vi "Process.vi"(9 "process sync":refnum<notifier>, 11 "Temp01 in":refnum<class "TELLC_Temp01.lvclass">) -> ()   [LabVIEW 2017, in "TELLC_Temp01.lvclass"]
doc: "Developed by Kevin Thompson\nkevin@thompsonengineering.net\n\nCopyright 2018\nThompson Engineering, LLC"
uses:
  TELLC_Temp01.lvclass
  DataTypes/Read Data--cluster.ctl
  DataTypes/Process - AppData--cluster.ctl
  DataTypes/Settings--cluster.ctl
  DataTypes/Dependency--cluster.ctl
  DataTypes/Public Events--cluster.ctl
  Common/DataTypes/TD Async CmdMsg EventData--cluster.ctl
  TELLC_Temp01.lvclass/TELLC_Temp01.ctl
  Accessors/Get Settings.vi
  Accessors/Get PublicEvents.vi
  Accessors/Get Dependency.vi
  <vilib>/TELLC/SMQ/Add States to Queue using MultiLine String with vData.vi
panel:
  out "Temp01ReadData":T1
  in  "Exit":bool
  # "local data monitoring"
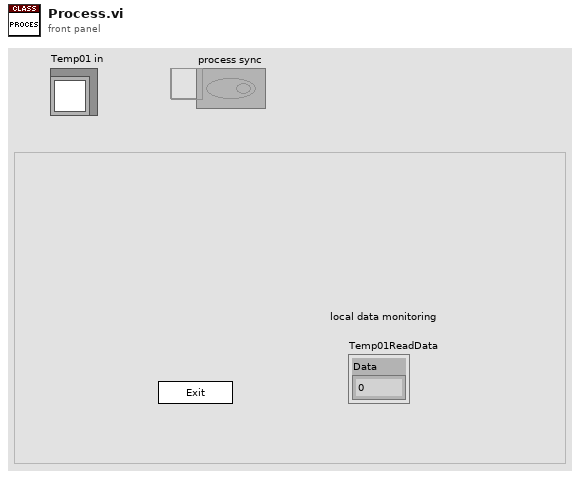
[diagram p1: front panel]
types:
  T1 = typedef "TELLC_Temp01.lvclass/Read Data--cluster.ctl" = cluster{"Data":dbl}
  T2 = typedef "TELLC_Temp01.lvclass/Process - AppData--cluster.ctl" = cluster{"Core":cluster{"Current VI Reference":refnum<vi>, "Close Panel on Exit?":bool}, "Your Boolean data":bool, "Your string data":string, "SMQ":refnum<queue>, "Initialized?":bool, "Self Reference":refnum<class "TELLC_Temp01.lvclass">, "Simulation?":bool, "process sync":refnum<notifier>, "vData":variant, "Settings":T3, "Dependency":T4, "Public Events":T5}
  T3 = typedef "TELLC_Temp01.lvclass/Settings--cluster.ctl" = cluster{"Simulation":bool}
  T4 = typedef "TELLC_Temp01.lvclass/Dependency--cluster.ctl" = cluster{"Config":refnum<class>, "ClassRef":refnum<class>}
  T5 = typedef "TELLC_Temp01.lvclass/Public Events--cluster.ctl" = cluster{"Temp01.AsyncCmd Event":refnum<user-event>, "Temp01.AsyncMsg Event":refnum<user-event>, "stop process":refnum<user-event>}
  T6 = enum32{"invalid app kind", "Development System", "Run Time System", "Student Edition", "Embedded LabVIEW", "Evaluation", "Custom"}
  T7 = enum32{"Invalid", "Standard", "Closed", "Hidden", "Minimized", "Maximized"}
  T8 = typedef "TELLC_Temp01.lvclass/AsynCmd_Temp01--enum.ctl" = enum16{"Temp01.DoSomething"}
  T9 = cluster{"Current VI Reference":refnum<vi>, "Close Panel on Exit?":bool}
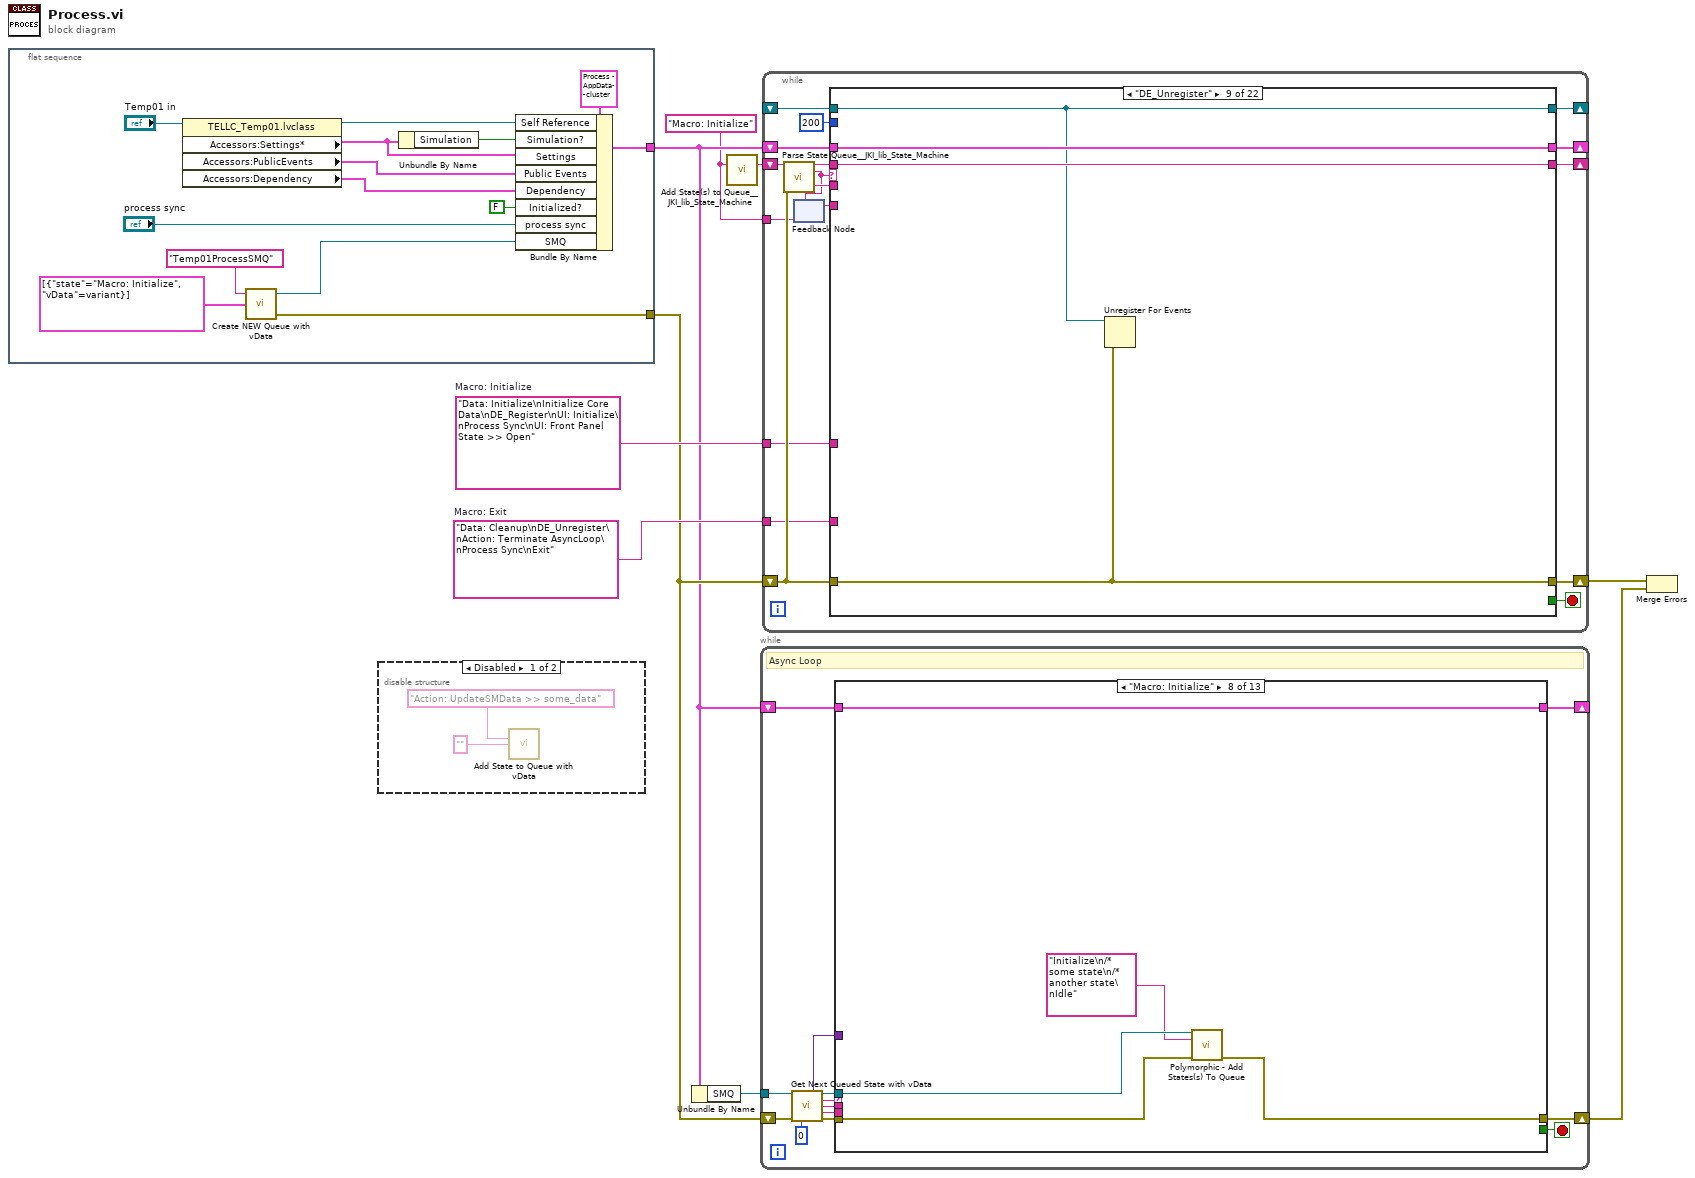
[diagram p0: block diagram]
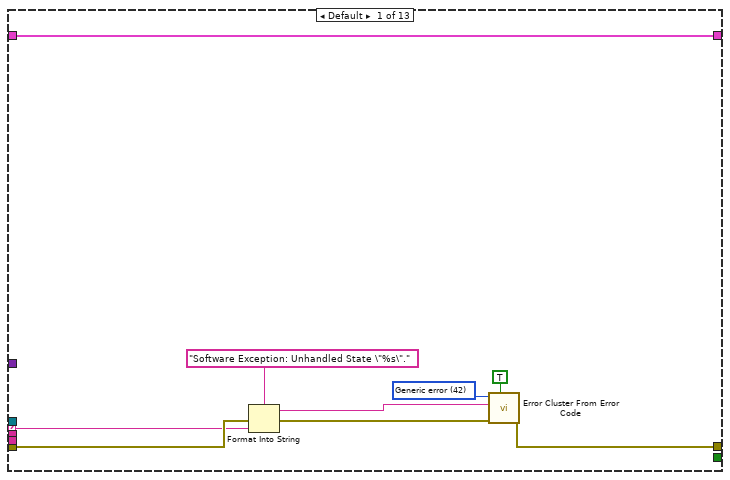
[diagram p3: hidden frame]
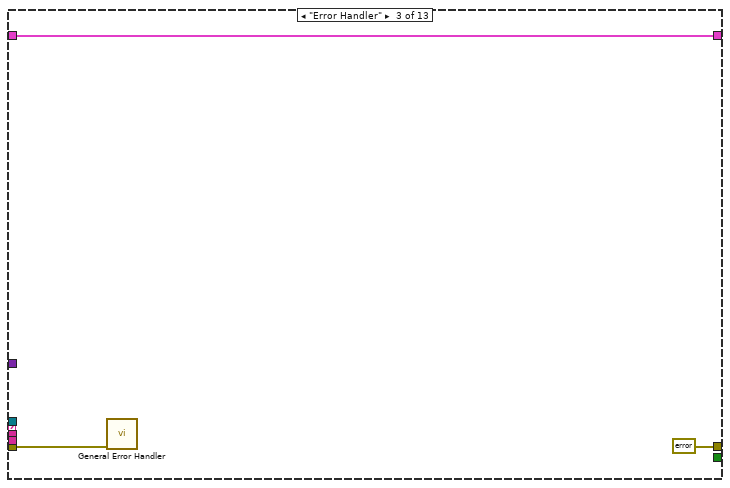
[diagram p5: hidden frame]
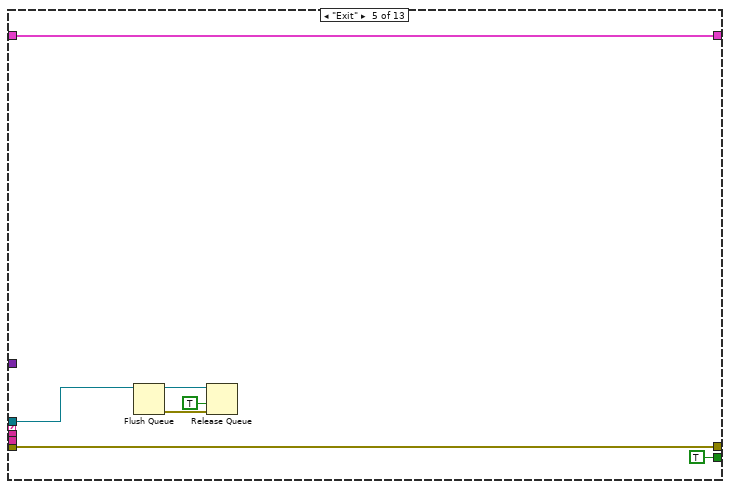
[diagram p7: hidden frame]
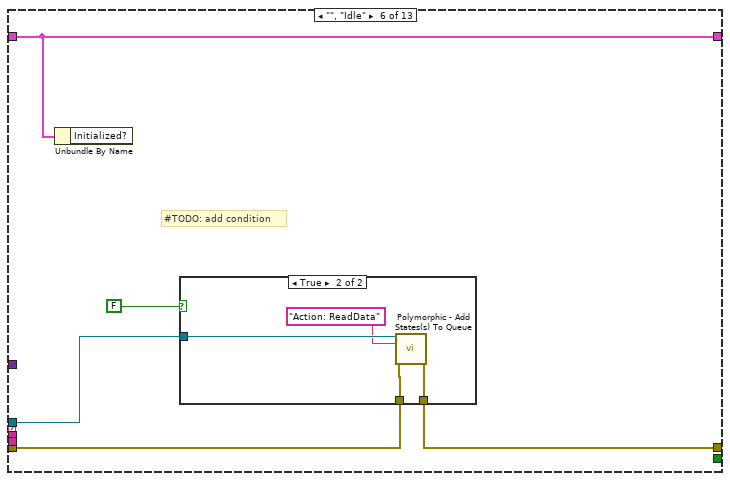
[diagram p8: hidden frame]
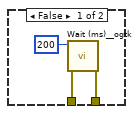
[diagram p9: hidden frame]
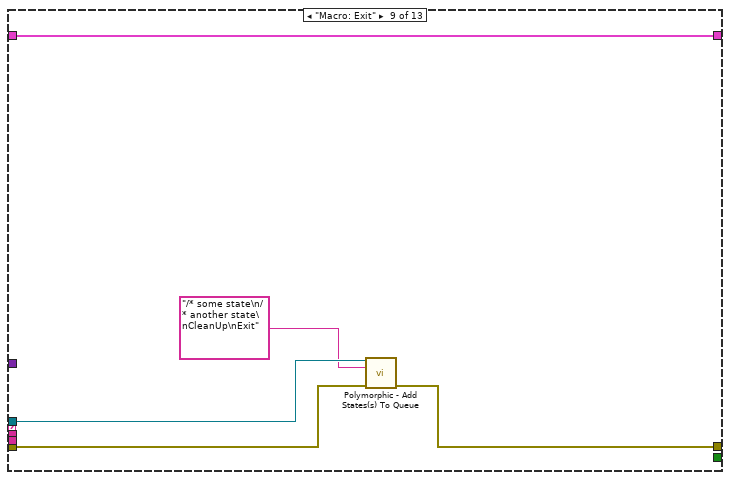
[diagram p11: hidden frame]
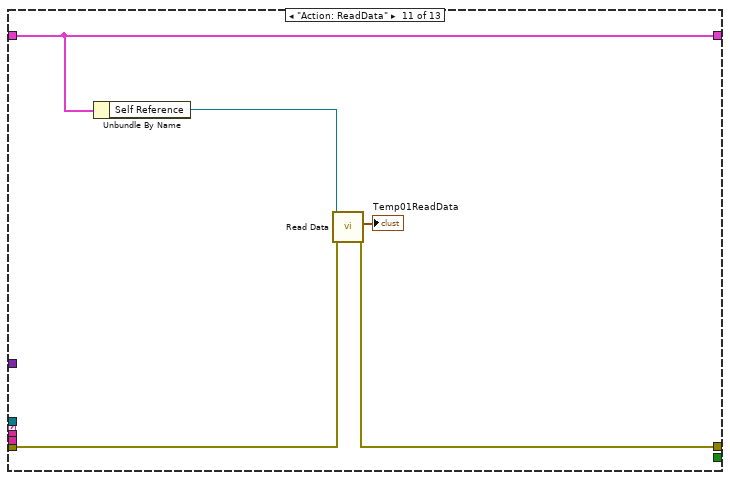
[diagram p13: hidden frame]
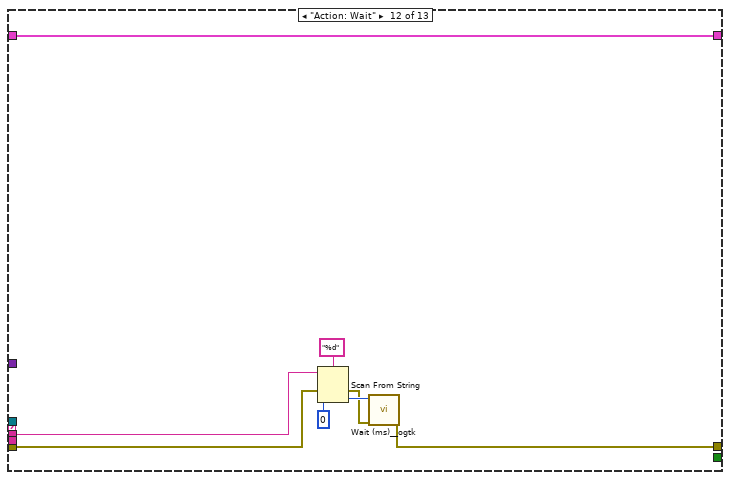
[diagram p14: hidden frame]
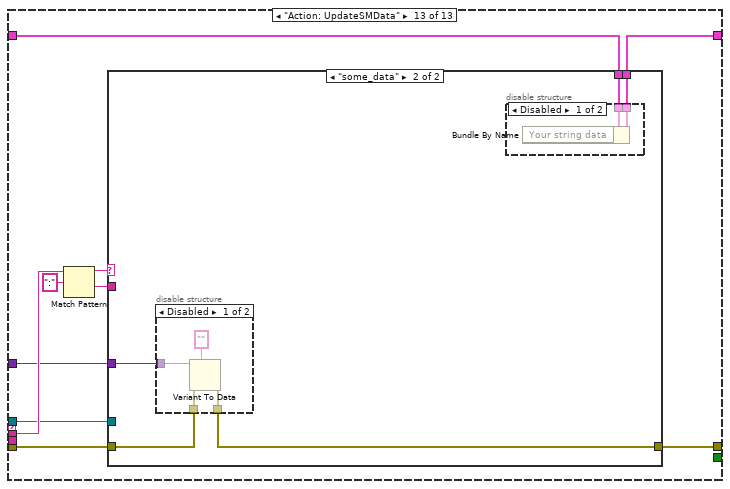
[diagram p15: hidden frame]
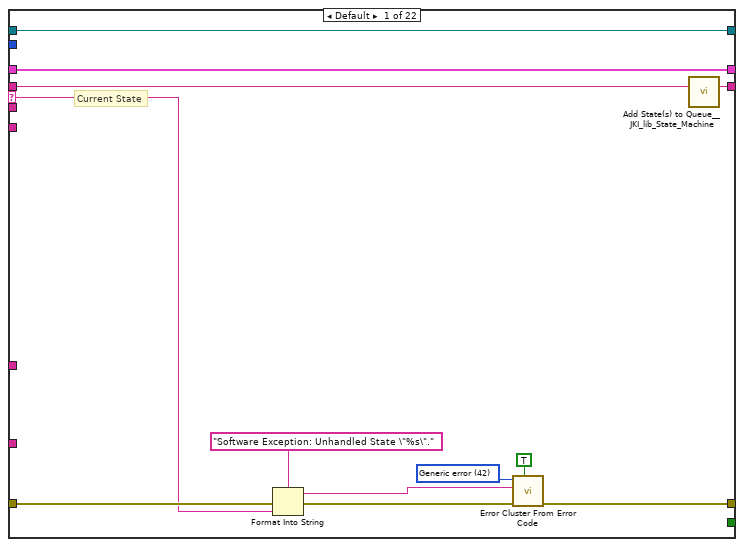
[diagram p19: hidden frame]
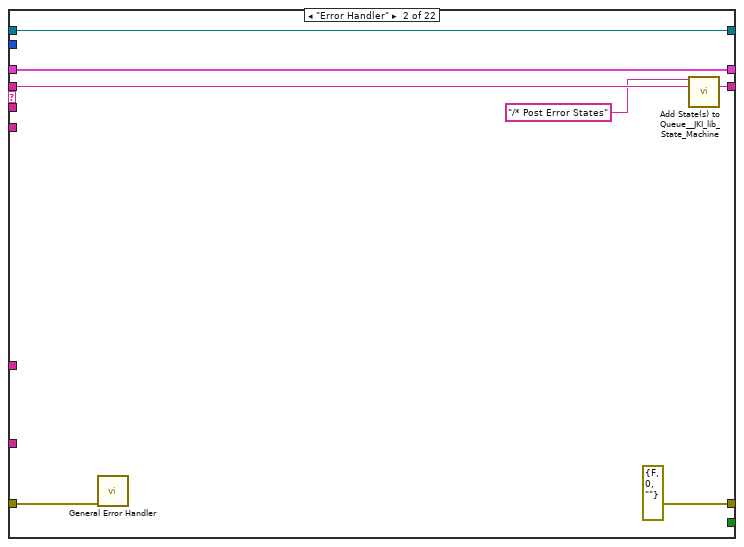
[diagram p20: hidden frame]
diagram:
  w7 = "Data: Cleanup\nDE_Unregister\nAction: Terminate AsyncLoop\nProcess Sync\nExit"  # Macro: Exit
  w8 = "Data: Initialize\nInitialize Core Data\nDE_Register\nUI: Initialize\nProcess Sync\nUI: Front Panel State >> Open"  # Macro: Initialize
  w1 = "Macro: Initialize"
  n1 = flat-sequence {
    tunnel: [w23] -> w4
    tunnel: [w20] -> w6
    frame #0 {
      n2 = property class="TELLC_Temp01.lvclass"(reference="Temp01 in") -> (reference out=w16:refnum<class "TELLC_Temp01.lvclass">, "Accessors:Settings*"=w11:T3, "Accessors:PublicEvents"=w13:T5, "Accessors:Dependency"=w14:T4)  [unwired: 1 in, 1 out]
      n3 = call <vilib>:"Create NEW Queue with vData.vi"("Initial States"=cluster{"state":string, "vData":variant}[] [{"state"="Macro: Initialize", "vData"=variant}], "Name (SMQ)"="Temp01ProcessSMQ") -> ("error out"=w20:errorcluster, "queue out"=w22:refnum<queue>)  [unwired: 2 in]
      n4 = Unbundle By Name(w11) -> ("Simulation"=w12:bool)
      n5 = Bundle By Name(cluster=T2 {"Core"={"Current VI Reference"=refnum, "Close Panel on Exit?"=FALSE}, "Your Boolean data"=FALSE, "Your string data"="", "SMQ"=refnum, "Initialized?"=FALSE, "Self Reference"=refnum, "Simulation?"=FALSE, "process sync"=refnum, "vData"=variant, "Settings"={"Simulation"=FALSE}, "Dependency"={"Config"=refnum, "ClassRef"=refnum}, "Public Events"={"Temp01.AsyncCmd Event"=refnum, "Temp01.AsyncMsg Event"=refnum, "stop process"=refnum}} ("SM2 AppData"), "Self Reference"=w16, "Simulation?"=w12, "Settings"=w11, "Public Events"=w13, "Dependency"=w14, "Initialized?"=FALSE, "process sync"="process sync", "SMQ"=w22) -> (w23:T2)
    }
  }
  n6 = disable-structure shown="Disabled" {
    frame Disabled {
      n7 = call <vilib>:"Add State to Queue with vData.vi"("state in"="Action: UpdateSMData >> some_data", "vData (\"\")"="") -> ()  [unwired: 10 in, 4 out]
    }
    frame Enabled {
    }
  }
  n8 = Unbundle By Name(w4) -> ("SMQ"=w5:refnum<queue>)
  n9 = call <vilib>:"Add State(s) to Queue__JKI_lib_State_Machine.vi"("State(s) in (\"\")"=w1) -> ("States Out"=w9:string)  [unwired: 14 in]
  n10 = while {
    shift-right: [w35] -> w2
    shift-left: w6 -> [w37]
    tunnel: w5 -> [w33]
    shift-right: [w31] -> _
    shift-left: w4 -> [w32]
    stop <- w26 stop-if-true
    # "Async Loop"
    n11 = call <vilib>:"Get Next Queued State with vData.vi"("queue in"=w33, "error in (no error)"=w37, "timeout (100)"=0) -> ("vData out"=w30:variant, "queue out"=w34:refnum<queue>, "Next State"=w38:string, "queued msg"=w28:string, "Prev State"=w27:string, "error out"=w36:errorcluster)  [unwired: 6 in, 1 out]
    n12 = case shown="\"Macro: Initialize\"" w38 {
      tunnel: w34 -> [_ _ _ _ w55 w63 _ w79 w84 _ _ _ w106]
      tunnel: w28 -> [_ _ _ _ _ _ _ _ _ _ _ w95 w108]
      selector: w38 -> [w39 _ _ _ _ _ _ _ _ _ _ _ _]
      tunnel: w36 -> [w41 w49 w50 w54 w61 w66 w75 w78 w83 w87 w90 w94 w103]
      tunnel: [w40 w49 errorcluster {"status"=FALSE, "code"=0, "source"=""} ("error constant") w54 w61 w65 w75 w77 w82 w87 w89 w97 w102] -> w35
      tunnel: w32 -> [w47 w48 w52 w53 w60 w62 w74 w80 w85 w86 w92 w100 w105]
      tunnel: [w47 w48 w52 w53 w60 w62 w74 w80 w85 w86 w92 w100 w104] -> w31
      tunnel: w30 -> [_ _ _ _ _ _ _ _ _ _ _ _ w107]
      tunnel: w27 -> [_ _ _ _ _ _ _ _ _ _ _ _ _]
      tunnel: [_ _ _ _ TRUE _ _ _ _ _ _ _ _] -> w26
      frame Default {
        w43 = 42 items=["No error", "Argument error", "Memory is full", "Out of zone", "End of file", "File already open", "Generic file I/O error", "File not found", "File permission error", "Disk is full", "Duplicate path", "Too many files open", "System feature not enabled", "Resource file not found", "Cannot add resource", "Resource not found", "Image not found", "Image memory error", "Pen does not exist", "Config type invalid", "Config token not found", "Config parse error", "Config memory error", "Bad external code format", "Bad external code offset", "External code not present", "Null window", "Destroy window error", "Null menu", "Print aborted", "Bad print record", "Print driver error", "Windows error during printing", "Memory error during printing", "Print dialog error", "Generic print error", "Invalid device refnum", "Device not found", "Device parameter error", "Device unit error", "Cannot open device", "Device call aborted", "Generic error", "Cancelled by user", "Object ID too low", "Object ID too high", "Object not in heap", "Unknown heap", "Unknown object (invalid DefProc)", "Unknown object (DefProc not in table)", "Message out of range", "Invalid (null) method", "Unknown message", "Manager call not supported", "Bad address", "Network operation in progress", "Network operation timed out", "Connection is busy", "Network attribute not supported", "Network error", "Address in use", "System out of memory", "Connection aborted", "Connection refused", "Not connected", "Already connected", "Connection closed", "Initialization error (interapplication manager)", "Bad occurrence", "Wait on unbound occurrence handler", "Occurrence queue overflow", "Datalog type conflict", "Unused", "Unrecognized type (interapplication manager)", "Memory corrupt", "Failed to make temporary DLL", "Old CIN version", "Drag socket not found", "Failed to load drop-object", "Failed to register OLE object", "Failed to release OLE object", "Format specifier type mismatch", "Unknown format specifier", "Too few format specifiers", "Too many format specifiers", "Scan failed", "Newer CIN version", "Error converting to variant", "Runtime menu error", "Password tampered", "Variant attribute not found", "Incompatible variant data type", "Event data is not available", "Event Store is not present", "Occurrence is not found", "Event Queue is not created", "Event info is not available", "Refnum passed is NULL", "Error retrieving Class GUID", "Error retrieving CoClass GUID", "Error retrieving TypeLib GUID.", "Bad built application magic bytes.", "Specific driver is different from the specific driver associated with the Logical Name.", "There is no session opened to the class driver.", "Max Error", "MAX - Error with config objects", "MAX - Error loading configuration", "MAX - Group not supported"]
        n13 = Format Into String(format string="Software Exception: Unhandled State \"%s\"." ("message"), error in=w41, w39) -> (resulting string=w44:string, error out=w45:errorcluster)  [unwired: 1 in]
        n14 = call <vilib>:"Error Cluster From Error Code.vi"("show call chain? (False)"=TRUE, "error in (no error)"=w45, "error message (\"\")"=w44, "error code (0)"=w43) -> ("error out"=w40:errorcluster)  [unwired: 5 in]
      }
      frame "Initialize" {
      }
      frame "Error Handler" {
        n15 = call <vilib>:"General Error Handler.vi"("error in (no error)"=w50) -> ()  [unwired: 10 in, 5 out]
      }
      frame "CleanUp" {
      }
      frame "Exit" {
        n16 = Flush Queue(queue=w55) -> (queue out=w58:refnum<queue>, error out=w57:errorcluster)  [unwired: 1 in, 1 out]
        n17 = Release Queue(queue=w58, force destroy? (F)=TRUE, error in (no error)=w57) -> ()  [unwired: 3 out]
      }
      frame "", "Idle" {
        # "#TODO: add condition"
        n18 = Unbundle By Name(w62) -> ()  [unwired: 1 out]
        n19 = case shown="True" FALSE {
          tunnel: w66 -> [w69 w73]
          tunnel: [w68 w72] -> w65
          tunnel: w63 -> [_ w71]
          frame False {
            n20 = call <userlib>:"Wait (ms)__ogtk.vi"("error in (no error)"=w69, "milliseconds to wait"=u32 200) -> ("error out"=w68:errorcluster)  [unwired: 8 in, 1 out]
          }
          frame True {
            n21 = call-poly <vilib>:"Polymorphic - Add States(s) To Queue.vi"("queue in"=w71, "state in"="Action: ReadData", "error in"=w73) -> ("error out"=w72:errorcluster)  [unwired: 9 in, 3 out]
          }
        }
      }
      frame "------ Macro ------" {
      }
      frame "Macro: Initialize" {
        n22 = call-poly <vilib>:"Polymorphic - Add States(s) To Queue.vi"("queue in"=w79, "states in"="Initialize\n/* some state\n/* another state\nIdle", "error in"=w78) -> ("error out"=w77:errorcluster)  [unwired: 10 in, 2 out]
      }
      frame "Macro: Exit" {
        n23 = call-poly <vilib>:"Polymorphic - Add States(s) To Queue.vi"("queue in"=w84, "states in"="/* some state\n/* another state\nCleanUp\nExit", "error in"=w83) -> ("error out"=w82:errorcluster)  [unwired: 10 in, 2 out]
      }
      frame "------ Action ------" {
      }
      frame "Action: ReadData" {
        n24 = Unbundle By Name(w92) -> ("Self Reference"=w91:refnum<class "TELLC_Temp01.lvclass">)
        n25 = call "Read Data.vi"("error in (no error)"=w90, "Temp01 in"=w91) -> ("error out"=w89:errorcluster, "Temp01ReadData"=→"Temp01ReadData":T1)  [unwired: 7 in, 1 out]
      }
      frame "Action: Wait" {
        n26 = Scan From String(format string="%d", input string=w95, error in=w94, default 1=u32 0) -> (error out=w93:errorcluster, output 1=w99:u32)  [unwired: 1 in, 2 out]
        n27 = call <userlib>:"Wait (ms)__ogtk.vi"("error in (no error)"=w93, "milliseconds to wait"=w99) -> ("error out"=w97:errorcluster)  [unwired: 8 in, 1 out]
      }
      frame "Action: UpdateSMData" {
        n28 = Match Pattern(string=w108, regular expression=":") -> (before substring=w110:string, after substring=w101:string)  [unwired: 1 in, 2 out]
        n29 = case shown="\"some_data\"" w110 {
          tunnel: w107 -> [_ w117]
          tunnel: w106 -> [_ _]
          tunnel: w105 -> [w111 w116]
          tunnel: [w111 w115] -> w104
          tunnel: w103 -> [w112 w114]
          tunnel: [w112 w113] -> w102
          tunnel: w101 -> [_ _]
          frame Default {
            # "#NOTE:\noptionally add error here."
          }
          frame "some_data" {
            n30 = disable-structure shown="Disabled" {
              disable-tunnel: w117 -> [w124 _]
              disable-tunnel: w114 -> [w122 w125]
              disable-tunnel: [w121 w125] -> w113
              frame Disabled {
                n31 = Variant To Data(error in=w122, type="", Variant=w124) -> (error out=w121:errorcluster)  [unwired: 1 out]
              }
              frame Enabled {
              }
            }
            n32 = disable-structure shown="Disabled" {
              disable-tunnel: w116 -> [w119 w120]
              disable-tunnel: [w118 w120] -> w115
              frame Disabled {
                n33 = Bundle By Name(cluster=w119) -> (w118:T2)  [unwired: 1 in]
              }
              frame Enabled {
              }
            }
          }
        }
      }
    }
  }
  n34 = while {
    shift-right: [w136] -> _
    shift-left: w4 -> [w135]
    shift-right: [w139] -> w3
    shift-left: w6 -> [w134]
    shift-right: [w138] -> _
    shift-left: w9 -> [w140]
    shift-right: [w133] -> _
    shift-left: _ -> [w132]
    tunnel: w8 -> [w130]
    tunnel: w7 -> [w129]
    tunnel: w1 -> [w128]
    stop <- w137 stop-if-true
    n35 = call <vilib>:"Parse State Queue__JKI_lib_State_Machine.vi"("State Queue"=w140, "Error In (no error)"=w134) -> ("Remaining States"=w142:string, "Current State"=w127:string, "Arguments"=w141:string)  [unwired: 11 in]
    n36 = feedback #1(w128) -> (w126:string)
    n37 = feedback-in #1(w127) -> ()
    n38 = case shown="\"DE_Unregister\"" w127 {
      selector: w127 -> [w144 _ _ _ _ _ _ _ _ _ _ _ _ _ _ _ _ _ _ _ _ _]
      tunnel: w142 -> [w148 w161 w167 w175 w238 w251 w259 w264 w268 w273 w282 w289 w294 w302 w311 w323 w350 w356 w367 w372 w383 w392]
      tunnel: w141 -> [_ _ _ _ _ _ _ _ _ _ _ _ _ _ w306 w317 _ _ _ _ w373 _]
      tunnel: w135 -> [w146 w158 w165 w173 w235 w242 w256 w261 w267 w270 w274 w284 w291 w297 w309 w319 w347 w353 w364 w369 w381 w389]
      tunnel: [w150 errorcluster {"status"=FALSE, "code"=0, "source"=""} ("error out") w164 w172 w236 w248 w252 w262 w265 w271 w280 w285 w292 w298 w307 w320 w348 w354 w365 w370 w374 w384] -> w139
      tunnel: w134 -> [w149 w157 w164 w171 w236 w248 w253 _ w265 w271 w280 w286 w292 w299 w308 w321 w348 w354 w365 w370 w375 w385]
      tunnel: [w147 w160 w166 w174 w237 w250 w258 w264 w268 w272 w281 w288 w293 w301 w310 w322 w349 w355 w366 w371 w382 w391] -> w138
      tunnel: [_ _ TRUE _ _ _ _ _ _ _ _ _ _ _ _ _ _ _ _ _ _ _] -> w137
      tunnel: [w146 w158 w165 w170 w235 w249 w256 w261 w267 w270 w276 w284 w291 w297 w309 w319 w347 w353 w364 w369 w381 w389] -> w136
      tunnel: [w143 w155 w162 w168 w234 w239 w257 w263 w266 w269 w275 w283 w290 w300 w305 w316 w346 w352 w358 w368 w380 w390] -> w133
      tunnel: w132 -> [w143 w155 w162 w168 w234 w239 w257 _ w266 w269 w275 w283 w290 w300 w305 w316 w346 w352 w358 w368 w380 w390]
      tunnel: 200 ("Timeout") -> [_ _ _ w169 _ _ _ _ _ _ _ _ _ _ _ _ _ _ _ _ _ _]
      tunnel: w130 -> [_ _ _ _ _ _ _ _ _ _ _ _ _ _ _ _ _ w351 _ _ _ _]
      tunnel: w129 -> [_ _ _ _ _ _ _ _ _ _ _ _ _ _ _ _ _ _ w357 _ _ _]
      tunnel: w126 -> [_ _ _ _ _ _ _ _ _ _ _ _ _ _ _ _ _ _ _ _ _ _]
      frame Default {
        w153 = 42 items=["No error", "Argument error", "Memory is full", "Out of zone", "End of file", "File already open", "Generic file I/O error", "File not found", "File permission error", "Disk is full", "Duplicate path", "Too many files open", "System feature not enabled", "Resource file not found", "Cannot add resource", "Resource not found", "Image not found", "Image memory error", "Pen does not exist", "Config type invalid", "Config token not found", "Config parse error", "Config memory error", "Bad external code format", "Bad external code offset", "External code not present", "Null window", "Destroy window error", "Null menu", "Print aborted", "Bad print record", "Print driver error", "Windows error during printing", "Memory error during printing", "Print dialog error", "Generic print error", "Invalid device refnum", "Device not found", "Device parameter error", "Device unit error", "Cannot open device", "Device call aborted", "Generic error", "Cancelled by user", "Object ID too low", "Object ID too high", "Object not in heap", "Unknown heap", "Unknown object (invalid DefProc)", "Unknown object (DefProc not in table)", "Message out of range", "Invalid (null) method", "Unknown message", "Manager call not supported", "Bad address", "Network operation in progress", "Network operation timed out", "Connection is busy", "Network attribute not supported", "Network error", "Address in use", "System out of memory", "Connection aborted", "Connection refused", "Not connected", "Already connected", "Connection closed", "Initialization error (interapplication manager)", "Bad occurrence", "Wait on unbound occurrence handler", "Occurrence queue overflow", "Datalog type conflict", "Unused", "Unrecognized type (interapplication manager)", "Memory corrupt", "Failed to make temporary DLL", "Old CIN version", "Drag socket not found", "Failed to load drop-object", "Failed to register OLE object", "Failed to release OLE object", "Format specifier type mismatch", "Unknown format specifier", "Too few format specifiers", "Too many format specifiers", "Scan failed", "Newer CIN version", "Error converting to variant", "Runtime menu error", "Password tampered", "Variant attribute not found", "Incompatible variant data type", "Event data is not available", "Event Store is not present", "Occurrence is not found", "Event Queue is not created", "Event info is not available", "Refnum passed is NULL", "Error retrieving Class GUID", "Error retrieving CoClass GUID", "Error retrieving TypeLib GUID.", "Bad built application magic bytes.", "Specific driver is different from the specific driver associated with the Logical Name.", "There is no session opened to the class driver.", "Max Error", "MAX - Error with config objects", "MAX - Error loading configuration", "MAX - Group not supported"]
        # "Current State"
        n39 = Format Into String(format string="Software Exception: Unhandled State \"%s\"." ("message"), error in=w149, w144) -> (resulting string=w152:string, error out=w151:errorcluster)  [unwired: 1 in]
        n40 = call <vilib>:"Error Cluster From Error Code.vi"("show call chain? (False)"=TRUE, "error in (no error)"=w151, "error message (\"\")"=w152, "error code (0)"=w153) -> ("error out"=w150:errorcluster)  [unwired: 5 in]
        n41 = call <vilib>:"Add State(s) to Queue__JKI_lib_State_Machine.vi"("State(s) in (\"\")"=w148) -> ("States Out"=w147:string)  [unwired: 14 in]
      }
      frame "Error Handler" {
        n42 = call <vilib>:"General Error Handler.vi"("error in (no error)"=w157) -> ()  [unwired: 10 in, 5 out]
        n43 = call <vilib>:"Add State(s) to Queue__JKI_lib_State_Machine.vi"("State(s) in Front (\"\")"="/* Post Error States", "State(s) in (\"\")"=w161) -> ("States Out"=w160:string)  [unwired: 13 in]
      }
      frame "Exit" {
        n44 = call <vilib>:"Add State(s) to Queue__JKI_lib_State_Machine.vi"("State(s) in (\"\")"=w167) -> ("States Out"=w166:string)  [unwired: 14 in]
      }
      frame "", "Event Structure", "Idle" {
        n45 = event shown="[5] <Public Events.Temp01.AsyncCmd Event>: User Event" {
          selector: w168 -> [_ _ _ _ _ _]
          dyn-events: _ -> [_ _ _ _ _ _]
          timeout: w169 -> [_ _ _ _ _ _]
          tunnel: w175 -> [w179 w184 w190 w193 w200 w216]
          tunnel: [w178 w183 w189 w192 w199 w215] -> w174
          tunnel: w173 -> [w176 w181 w187 w195 w203 w205]
          tunnel: [w177 w182 w188 w196 w204 w213] -> w172
          tunnel: w171 -> [w177 w182 w188 w196 w204 w212]
          tunnel: [w176 w181 w187 w195 w202 w207] -> w170
          event Timeout {
            n46 = event-data() -> ()  [unwired: 1 in, 1 out]
            n47 = call <vilib>:"Add State(s) to Queue__JKI_lib_State_Machine.vi"("State(s) in (\"\")"=w179) -> ("States Out"=w178:string)  [unwired: 14 in]
          }
          event "Exit": Value Change {
            n48 = event-data() -> ()  [unwired: 1 in, 1 out]
            n49 = call <vilib>:"Add State(s) to Queue__JKI_lib_State_Machine.vi"("State(s) in Front (\"\")"="Macro: Exit", "State(s) in (\"\")"=w184) -> ("States Out"=w183:string)  [unwired: 13 in]
          }
          event Panel Close? {
            n50 = event-data() -> ()  [unwired: 1 in, 1 out]
            n51 = event-data("Discard?"=TRUE) -> ()  [unwired: 1 in, 1 out]
            n52 = call <vilib>:"Add State(s) to Queue__JKI_lib_State_Machine.vi"("State(s) in Front (\"\")"="Macro: Exit", "State(s) in (\"\")"=w190) -> ("States Out"=w189:string)  [unwired: 13 in]
          }
          event Menu Selection (User) {
            n53 = event-data() -> ("ItemTag"=w194:string)  [unwired: 1 in, 2 out]
            n54 = case shown="\"False\", Default" w194 {
              tunnel: [""] -> w191
              frame "False", Default {
              }
            }
            n55 = call <vilib>:"Add State(s) to Queue__JKI_lib_State_Machine.vi"("State(s) in Front (\"\")"=w191, "State(s) in (\"\")"=w193) -> ("States Out"=w192:string)  [unwired: 13 in]
          }
          event User Event {
            n56 = event-data() -> ("notifier out"=w201:refnum<notifier>)  [unwired: 1 in]
            n57 = Bundle By Name(cluster=w203, "process sync"=w201) -> (w202:T2)
            n58 = call <vilib>:"Add State(s) to Queue__JKI_lib_State_Machine.vi"("State(s) in Front (\"\")"="Macro: Exit", "State(s) in (\"\")"=w200) -> ("States Out"=w199:string)  [unwired: 13 in]
          }
          event User Event {
            n59 = event-data() -> ("CmdMsg"=w210:string, "vData"=w214:variant)  [unwired: 1 in, 1 out]
            n60 = Unbundle By Name(w205) -> ("Self Reference"=w206:refnum<class "TELLC_Temp01.lvclass">)
            n61 = call "get async cmd.vi"("error in (no error)"=w212, "Cmd String in"=w210) -> ("error out"=w211:errorcluster, "AsyncCmd"=w209:T8)  [unwired: 8 in]
            n62 = case shown="\"Temp01.DoSomething\"" w209 {
              tunnel: w214 -> [_ w229]
              tunnel: w211 -> [w222 w228]
              tunnel: [w221 w227] -> w213
              tunnel: [_ ""] -> w208
              tunnel: w205 -> [w217 w225]
              tunnel: [w217 w224] -> w207
              tunnel: w206 -> [_ _]
              tunnel: w205 -> [_ _]
              frame Default {
                n63 = call <vilib>:"Build Error Cluster_ModKT .vi"("Prepend String (\"\")"="Invalid Async Cmd" ("Prepend String (\"\")"), "code"=42, "error? (F)"=TRUE, "error in (no error)"=w222) -> ("error out"=w221:errorcluster)  [unwired: 3 in, 1 out]
              }
              frame "Temp01.DoSomething" {
                n64 = disable-structure shown="Disabled" {
                  disable-tunnel: w229 -> [w232 _]
                  disable-tunnel: w228 -> [w231 w233]
                  disable-tunnel: [w230 w233] -> w227
                  frame Disabled {
                    n65 = Variant To Data(error in=w231, Variant=w232) -> (error out=w230:errorcluster)  [unwired: 1 in, 1 out]
                  }
                  frame Enabled {
                  }
                }
                n66 = Bundle By Name(cluster=w225, "vData"=variant) -> (w224:T2)
              }
            }
            n67 = call <vilib>:"Add State(s) to Queue__JKI_lib_State_Machine.vi"("State(s) in Front (\"\")"=w208, "State(s) in (\"\")"=w216) -> ("States Out"=w215:string)  [unwired: 13 in]
          }
        }
      }
      frame "---------- Core ----------" {
        n68 = call <vilib>:"Add State(s) to Queue__JKI_lib_State_Machine.vi"("State(s) in (\"\")"=w238) -> ("States Out"=w237:string)  [unwired: 14 in]
      }
      frame "Initialize Core Data" {
        # "originally closed?"
        # "exe?"
        n69 = property class="VI"() -> ("Front Panel.Open"=w247:bool)  [unwired: 2 in, 2 out]
        n70 = property class="App"() -> ("App.Kind"=w246:T6)  [unwired: 2 in, 2 out]
        n71 = control-ref of="Current VI Reference"() -> (w240:refnum<vi>)
        n72 = Not(x=w247) -> (.not. x?=w244:bool)
        n73 = Equal?(x=w246, y=T6."Run Time System" ("Application:Kind")) -> (x = y?=w243:bool)
        n74 = Or(x=w244, y=w243) -> (x .or. y?=w241:bool)
        n75 = Bundle By Name(cluster=w242, "Core.Current VI Reference"=w240, "Core.Close Panel on Exit?"=w241) -> (w249:T2)
        n76 = call <vilib>:"Add State(s) to Queue__JKI_lib_State_Machine.vi"("State(s) in (\"\")"=w251) -> ("States Out"=w250:string)  [unwired: 14 in]
      }
      frame "Process Sync" {
        n77 = Unbundle By Name(w256) -> ("process sync"=w255:refnum<notifier>)
        n78 = Send Notification(notification=TRUE, notifier=w255, error in (no error)=w253) -> (error out=w252:errorcluster)  [unwired: 1 out]
        n79 = call <vilib>:"Add State(s) to Queue__JKI_lib_State_Machine.vi"("State(s) in (\"\")"=w259) -> ("States Out"=w258:string)  [unwired: 14 in]
      }
      frame "DE_Register" {
        n80 = Unbundle By Name(w261) -> ("Public Events"=w260:T5)
        n81 = register-events(w260) -> (reference out=w263:refnum<event-registration>, error out=w262:errorcluster)  [unwired: 2 in]
      }
      frame "DE_Unregister" {
        n82 = Unregister For Events(event registration refnum=w266, error in=w265) -> ()  [unwired: 1 out]
      }
      frame "---------- Data ----------" {
        n83 = call <vilib>:"Add State(s) to Queue__JKI_lib_State_Machine.vi"("State(s) in (\"\")"=w273) -> ("States Out"=w272:string)  [unwired: 14 in]
      }
      frame "Data: Initialize" {
        w277 = T9 {"Current VI Reference"=refnum, "Close Panel on Exit?"=FALSE}  # Core
        w279 = TRUE  # Your Boolean data
        w278 = ""  # Your string data
        n84 = Unbundle By Name(w274) -> ()  [unwired: 1 out]
        n85 = Bundle By Name(cluster=w274, "Core"=w277, "Your Boolean data"=w279, "Your string data"=w278) -> (w276:T2)
        n86 = call <vilib>:"Add State(s) to Queue__JKI_lib_State_Machine.vi"("State(s) in (\"\")"=w282) -> ("States Out"=w281:string)  [unwired: 14 in]
      }
      frame "Data: Cleanup" {
        n87 = Unbundle By Name(w284) -> ("Core.Current VI Reference"=w287:refnum<vi>)
        n88 = Close Reference(reference=w287, error in (no error)=w286) -> (error out=w285:errorcluster)
        n89 = call <vilib>:"Add State(s) to Queue__JKI_lib_State_Machine.vi"("State(s) in (\"\")"=w289) -> ("States Out"=w288:string)  [unwired: 14 in]
      }
      frame "---------- UI ----------" {
        n90 = call <vilib>:"Add State(s) to Queue__JKI_lib_State_Machine.vi"("State(s) in (\"\")"=w294) -> ("States Out"=w293:string)  [unwired: 14 in]
      }
      frame "UI: Initialize" {
        n91 = Unbundle By Name(w297) -> ("Core.Current VI Reference"=w296:refnum<vi>)
        n92 = call <userlib>:"Fit VI window to Largest Dec__ogtk.vi"("error in (no error)"=w299, "VI Ref (calling VI)"=w296) -> ("error out"=w298:errorcluster, "dup VI Ref"=w295:refnum<vi>)  [unwired: 4 in]
        n93 = disable-structure shown="Disabled" {
          disable-tunnel: w295 -> [w304 _]
          frame Disabled {
            n94 = property class="VI"(reference=w304, "Front Panel.Title"="*VI Title*" ("Front Panel Window:Title")) -> ()  [unwired: 1 in, 2 out]
          }
          frame Enabled {
          }
        }
        n95 = call <vilib>:"Add State(s) to Queue__JKI_lib_State_Machine.vi"("State(s) in (\"\")"=w302) -> ("States Out"=w301:string)  [unwired: 14 in]
      }
      frame "UI: Cursor Set" {
        # "Argument"
        n96 = case shown="\"Idle\", Default" w306 {
          tunnel: w308 -> [w313 w315]
          tunnel: [w312 w314] -> w307
          frame "Idle", Default {
            n97 = call <vilib>:"Unset Busy.vi"("error in (no error)"=w313) -> ("error out"=w312:errorcluster)  [unwired: 10 in]
          }
          frame "Busy" {
            n98 = call <vilib>:"Set Busy.vi"("error in (no error)"=w315) -> ("error out"=w314:errorcluster)  [unwired: 9 in, 1 out]
          }
        }
        n99 = call <vilib>:"Add State(s) to Queue__JKI_lib_State_Machine.vi"("State(s) in (\"\")"=w311) -> ("States Out"=w310:string)  [unwired: 14 in]
      }
      frame "UI: Front Panel State" {
        # "Argument"
        n100 = Unbundle By Name(w319) -> ("Core.Current VI Reference"=w318:refnum<vi>)
        n101 = case shown="\"Close\"" w317 {
          tunnel: w321 -> [w327 w340]
          tunnel: [w329 w341] -> w320
          tunnel: w318 -> [w328 w338]
          frame "Open", Default {
            n102 = property class="VI"(reference=w328, error in=w327) -> (reference out=w325:refnum<vi>, error out=w326:errorcluster, "Front Panel.Open"=w324:bool)
            n103 = case shown="False" w324 {
              tunnel: [w332 w335] -> w329
              tunnel: w326 -> [w331 w335]
              tunnel: w325 -> [w330 _]
              frame False {
                n104 = invoke class="VI" method="FP.Open"(reference=w330, error in=w331, "Activate"=TRUE, "State"=T7."Standard") -> (error out=w332:errorcluster)  [unwired: 1 in, 4 out]
              }
              frame True {
              }
            }
          }
          frame "Close" {
            n105 = property class="VI"(reference=w338, error in=w340) -> (reference out=w337:refnum<vi>, error out=w339:errorcluster, "Front Panel.Open"=w336:bool)
            n106 = case shown="True" w336 {
              tunnel: [w342 w345] -> w341
              tunnel: w339 -> [w342 w344]
              tunnel: w337 -> [_ w343]
              frame False {
              }
              frame True {
                n107 = invoke class="VI" method="FP.Close"(reference=w343, error in=w344) -> (error out=w345:errorcluster)  [unwired: 1 in, 2 out]
              }
            }
          }
        }
        n108 = call <vilib>:"Add State(s) to Queue__JKI_lib_State_Machine.vi"("State(s) in (\"\")"=w323) -> ("States Out"=w322:string)  [unwired: 14 in]
      }
      frame "---------- Macro ----------" {
        n109 = call <vilib>:"Add State(s) to Queue__JKI_lib_State_Machine.vi"("State(s) in (\"\")"=w350) -> ("States Out"=w349:string)  [unwired: 14 in]
      }
      frame "Macro: Initialize" {
        n110 = call <vilib>:"Add State(s) to Queue__JKI_lib_State_Machine.vi"("State(s) in Front (\"\")"=w351, "State(s) in (\"\")"=w356) -> ("States Out"=w355:string)  [unwired: 13 in]
      }
      frame "Macro: Exit" {
        n111 = Unbundle By Name(w364) -> ("Core.Close Panel on Exit?"=w363:bool)
        n112 = Select(t="UI: Front Panel State >> Close", s=w363, f="") -> (s? t:f=w360:string)
        n113 = call <vilib>:"Add State(s) to Queue__JKI_lib_State_Machine.vi"("State(s) in (\"\")"=w360, "State(s) at Back (\"\")"=w357) -> ("States Out"=w359:string)  [unwired: 13 in]
        n114 = call <vilib>:"Add State(s) to Queue__JKI_lib_State_Machine.vi"("State(s) in Front (\"\")"=w359, "State(s) in (\"\")"=w367) -> ("States Out"=w366:string)  [unwired: 13 in]
      }
      frame "---------- Action ----------" {
        n115 = call <vilib>:"Add State(s) to Queue__JKI_lib_State_Machine.vi"("State(s) in (\"\")"=w372) -> ("States Out"=w371:string)  [unwired: 14 in]
      }
      frame "Action: Wait" {
        n116 = Scan From String(format string="%d", input string=w373, error in=w375, default 1=u32 0) -> (error out=w379:errorcluster, output 1=w378:u32)  [unwired: 1 in, 2 out]
        n117 = call <userlib>:"Wait (ms)__ogtk.vi"("error in (no error)"=w379, "milliseconds to wait"=w378) -> ("error out"=w374:errorcluster)  [unwired: 8 in, 1 out]
        n118 = call <vilib>:"Add State(s) to Queue__JKI_lib_State_Machine.vi"("State(s) in (\"\")"=w383) -> ("States Out"=w382:string)  [unwired: 14 in]
      }
      frame "Action: Terminate AsyncLoop" {
        n119 = Unbundle By Name(w389) -> ("SMQ"=w388:refnum<queue>)
        n120 = Flush Queue(queue=w388) -> (queue out=w387:refnum<queue>)  [unwired: 1 in, 2 out]
        n121 = call <vilib>:"Add State to Queue with vData.vi"("queue in"=w387, "state in"="Macro: Exit", "error in"=w385) -> ("error out"=w384:errorcluster)  [unwired: 9 in, 3 out]
        n122 = call <vilib>:"Add State(s) to Queue__JKI_lib_State_Machine.vi"("State(s) in (\"\")"=w392) -> ("States Out"=w391:string)  [unwired: 14 in]
      }
    }
  }
  n123 = Merge Errors(w3, w2) -> ()  [unwired: 1 out]
